vi "LINX - PmodTC1.vi"() -> ()   [LabVIEW 2019]
doc: "PmodTC1\n\nThis example demonstrates how to read the thermocouple and reference temperatures from the PmodTC1.\n\nInstructions:\n1. Select the COM Port associated with the LINX device\n2. Select the SPI Channel that the Pmod is connected to.\n3. Select the CS Channel that the Pmod is connected to.\n4. Click the Run Arrow."
uses:
  <vilib>/MakerHub/LINX/LMH-LINX.lvlib
  <vilib>/MakerHub/LINX/Public/Sensors/Pmods/TC1/PmodTC1.lvlib
panel:
  out "Waveform Chart":T1(graph)
  in  "Stop Button":bool
  out "Temperatures":T2
  in  "CS Channel":u8=10
  in  "SPI Channel (0)":u8
  in  "Serial Port":refnum<visa-resource-name>="N/A"
  # "PmodTC1\n\nThis example demonstrates how to read the thermocouple and reference temperatures from the PmodTC1.\n\nInstructions:\n1. Select the COM Port associated with the LINX device\n2. Select the SPI Channel that the Pmod is connected to.\n3. Select the CS Channel that the Pmod is connected to.\n4. Click the Run Arrow."
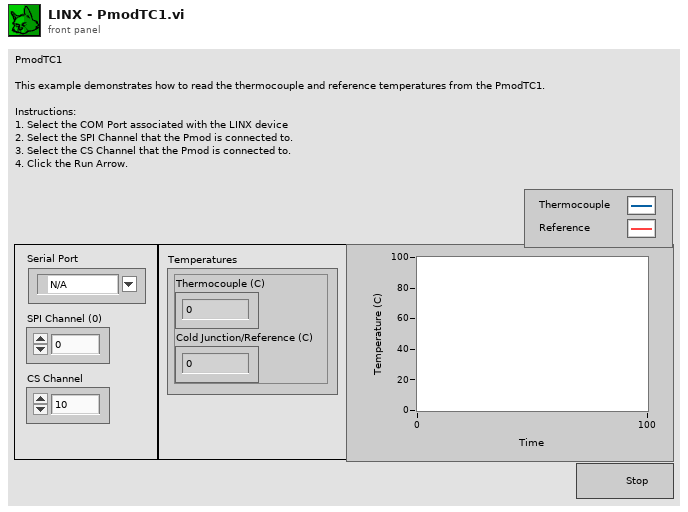
[diagram p1: front panel]
types:
  T1 = cluster{"Cold Junction (C)":i16, "Thermocouple (C)":i16}
  T2 = cluster{"Thermocouple (C)":i16, "Cold Junction/Reference (C)":i16}
  T3 = typedef "LMH-LINX.lvlib/LINX Ref.ctl" = cluster{"IO":T4, "Interface":T5, "LINX Device Config":T6}
  T4 = typedef "LMH-LINX.lvlib/Platform.ctl" = enum16{"Remote", "Local"}
  T5 = typedef "LMH-LINX.lvlib/Interface.ctl" = enum16{"Serial", "TCP"}
  T6 = typedef "LMH-LINX.lvlib/Device.lvlib/LINX Device Config.ctl" = cluster{"Interface":T5, "COM Port":refnum<visa-resource-name>, "TCP Configuration":T7, "Device Family":u8, "Device ID":u8, "Device Name":string, "TCP Ref":refnum<k5>, "Channels":T8}
  T7 = typedef "LMH-LINX.lvlib/Device.lvlib/TCP Config.ctl" = cluster{"IP Address":string, "Port":u16}
  T8 = typedef "LMH-LINX.lvlib/Channels.ctl" = cluster{"DI":u8[], "DO":u8[], "AI":u8[], "AO":u8[], "PWM":u8[], "QE":u8[], "UART":u8[], "I2C 2":u8[], "SPI":u8[], "CAN":u8[], "Servo":u8[], "AI Ref (V)":dbl, "AI Resolution (Bits)":u8, "AO Ref (V)":dbl, "AO Resolution (Bits)":u8}
  T9 = cluster{"Thermocouple (C)":i16, "Cold Junction (C)":i16}
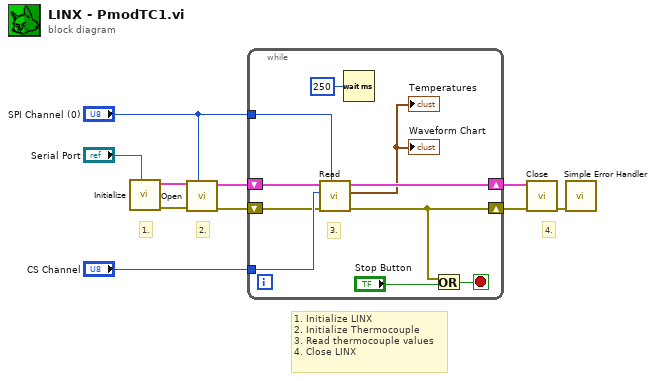
[diagram p0: block diagram]
diagram:
  # "1. Initialize LINX\n2. Initialize Thermocouple\n3. Read thermocouple values\n4. Close LINX"
  # "4."
  # "2."
  # "1."
  n1 = call <vilib>:"Initialize.vi"("Serial Port"="Serial Port") -> ("Error Out"=w5:errorcluster, "LINX Resource"=w6:T3)  [unwired: 8 in, 1 out]
  n2 = call <vilib>:"Open.vi"("SPI Channel (0)"="SPI Channel (0)", "Error In"=w5, "LINX Resource"=w6) -> ("Error Out"=w3:errorcluster, "LINX Resource"=w4:T3)  [unwired: 7 in]
  n3 = while {
    tunnel: "CS Channel" -> [w20]
    tunnel: "SPI Channel (0)" -> [w19]
    shift-right: [w16] -> w2
    shift-left: w4 -> [w18]
    shift-right: [w14] -> w1
    shift-left: w3 -> [w17]
    stop <- w13 stop-if-true
    # "3."
    n4 = call <vilib>:"Read.vi"("SPI Channel (0)"=w19, "Error In"=w17, "CS Channel"=w20, "LINX Resource"=w18) -> ("Error Out"=w14:errorcluster, "Temperatures"=→"Temperatures" →"Waveform Chart":T9, "LINX Resource"=w16:T3)  [unwired: 5 in]
    n5 = Wait (ms)(milliseconds to wait=u32 250) -> ()  [unwired: 1 out]
    n6 = Or(x=w14, y="Stop Button") -> (x .or. y?=w13:bool)
  }
  n7 = call <vilib>:"Close.vi"("Error In"=w1, "LINX Resource"=w2) -> ("Error Out"=w9:errorcluster)  [unwired: 9 in]
  n8 = call <vilib>:"Simple Error Handler.vi"("error in (no error)"=w9) -> ()  [unwired: 4 in, 5 out]
